vi "Ivdda_insert_db.vi"(11 "Array":string[](array[string])) -> (2 "String 2":string, 3 "ExitCode":i32)   [LabVIEW 2023]
uses:
  <vilib>/Utility/file.llb/Read Delimited Spreadsheet (string).vi
  <vilib>/addons/database/Connection.llb/DB Tools Open Connec (String).vi
  <vilib>/addons/database/NI_Database_API.lvlib
panel:
  out "cluster":T1
  out "error out":errorcluster
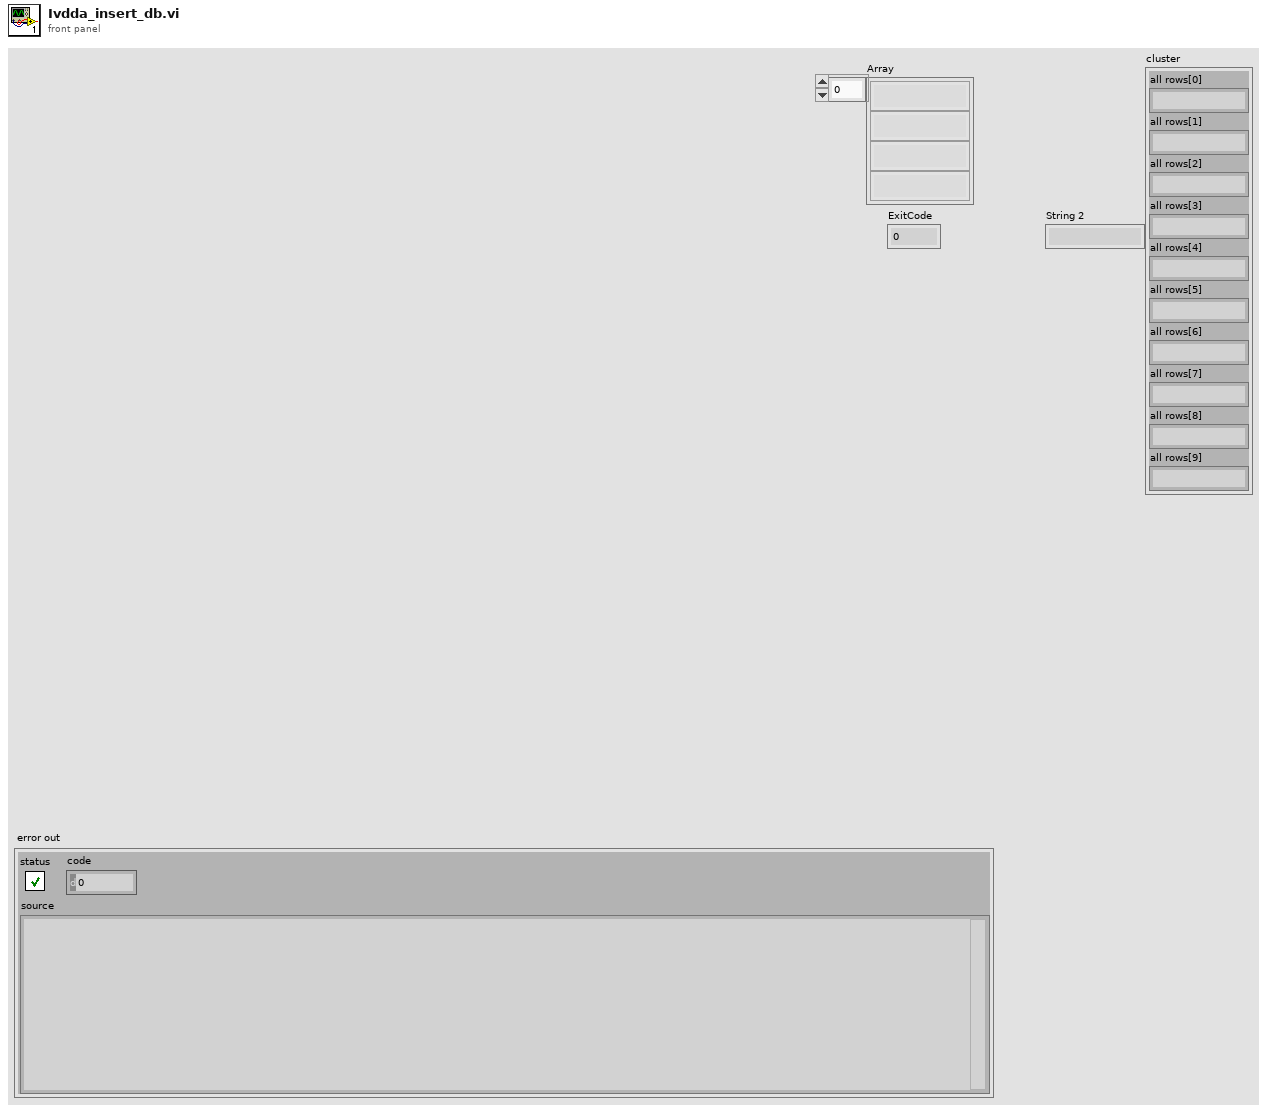
[diagram p1: front panel]
types:
  T1 = cluster{"all rows[0]":string, "all rows[1]":string, "all rows[2]":string, "all rows[3]":string, "all rows[4]":string, "all rows[5]":string, "all rows[6]":string, "all rows[7]":string, "all rows[8]":string, "all rows[9]":string}
  T2 = typedef "NI_Database_API.lvlib/Conn ObjectReference.ctl" = refnum<k1>
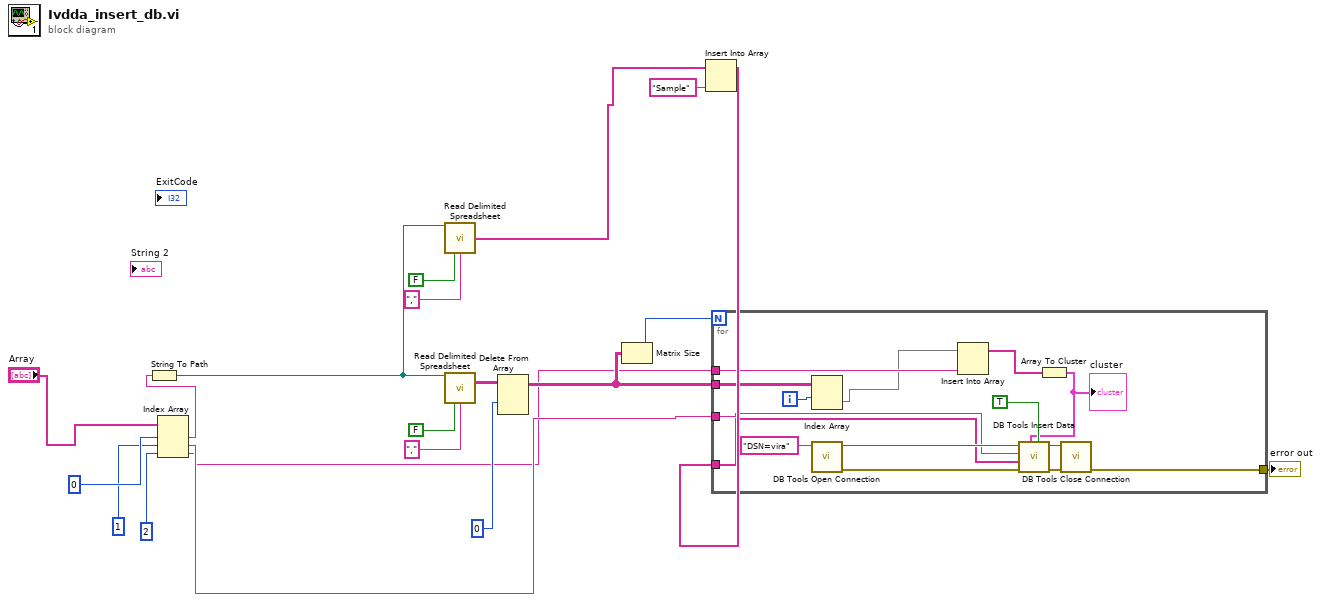
[diagram p0: block diagram]
diagram:
  n1 = Index Array(array="Array", index #1=0 ("index"), index #2=1 ("index"), index #3=2 ("index")) -> (element #1=w9:string, element #2=w7:string, element #3=w4:string)
  n2 = String To Path(string=w9) -> (path=w12:path)
  n3 = call-poly <vilib>:"Read Delimited Spreadsheet.vi"("file path (dialog if empty)"=w12, "transpose? (F)"=FALSE, "delimiter (\\t)"="," ("delimiter (\\t)")) -> ("first row"=w3:string[])  [unwired: 7 in, 5 out]
  n4 = call-poly <vilib>:"Read Delimited Spreadsheet.vi"("file path (dialog if empty)"=w12, "transpose? (F)"=FALSE, "delimiter (\\t)"="," ("delimiter (\\t)")) -> ("all rows"=w13:string[][])  [unwired: 7 in, 5 out]
  n5 = Delete From Array "Delete From Array"(array=w13, index (row)=0) -> (array with subset deleted=w5:string[][])  [unwired: 2 in, 1 out]
  n6 = Matrix Size(0:w5) -> (1:w20:i32)  [unwired: 1 out]
  n7 = Insert Into Array(array=w3, new element="Sample" ("new element/subarray")) -> (w1:string[])  [unwired: 1 in]
  n8 = for {
    N: w20 -> [_]
    tunnel: w5 -> [w34]
    tunnel: w1 -> [w27]
    tunnel: w7 -> [w26]
    tunnel: [w25] -> w19
    tunnel: w4 -> [w24]
    i -> [w35]
    n9 = Index Array "Index Array"(array=w34, index (row)=w35) -> (element=w23:string[])  [unwired: 1 in]
    n10 = call-poly <vilib>:"DB Tools Open Connection.vi"("connection information"="DSN=vira") -> ("error out"=w32:errorcluster, "connection reference"=w31:T2)  [unwired: 7 in]
    n11 = Insert Into Array "Insert Into Array"(array=w23, new element=w24) -> (w22:string[])  [unwired: 1 in]
    n12 = Array To Cluster(array=w22) -> (cluster=w21:T1)
    "cluster" <- w21
    n13 = call <vilib>:"DB Tools Insert Data.vi"("create table? (F)"=TRUE, "data"=w21, "error in (no error)"=w32, "columns"=w27, "table"=w26, "connection reference"=w31) -> ("error out"=w30:errorcluster, "connection reference out"=w29:T2)  [unwired: 4 in]
    n14 = call <vilib>:"DB Tools Close Connection.vi"("error in (no error)"=w30, "connection reference"=w29) -> ("error out"=w25:errorcluster)  [unwired: 5 in]
  }
  "error out" <- w19
